vi "Is Calling VI Running.vi"(8 "Error In":errorcluster, 11 "Calling VI Path":path) -> (0 "Error Out":errorcluster, 3 "Running?":bool)   [LabVIEW 2021, in "Notebook.lvlib"]
uses:
  Notebook.lvlib
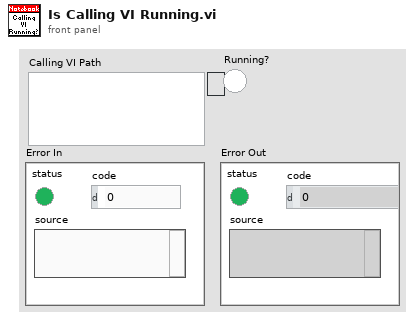
[diagram p1: front panel]
types:
  T1 = enum32{"Bad", "Idle", "Run top level", "Running"}[]
  T2 = enum32{"Invalid", "Standard", "Closed", "Hidden", "Minimized", "Maximized"}[]
  T3 = enum32{"Invalid", "Standard", "Closed", "Hidden", "Minimized", "Maximized"}
  T4 = enum32{"Bad", "Idle", "Run top level", "Running"}
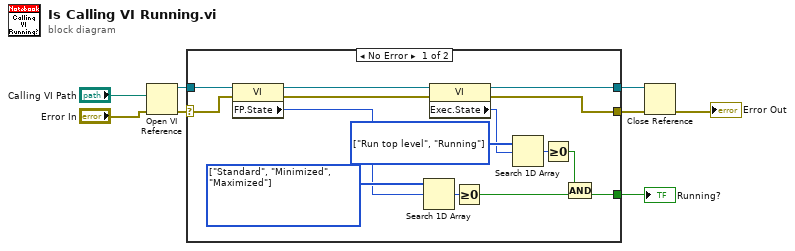
[diagram p0: block diagram]
diagram:
  n1 = Open VI Reference(vi path="Calling VI Path", error in (no error)="Error In") -> (vi reference=w8:refnum<vi>, error out=w6:errorcluster)  [unwired: 4 in]
  n2 = case shown="No Error" w6 {
    selector: w6 -> [w22 w24]
    tunnel: w8 -> [w23 w25]
    tunnel: [w14 w25] -> w7
    tunnel: [w16 w24] -> w5
    tunnel: [w10 _] -> w3
    frame No Error {
      w12 = T1 [enum."Run top level", enum."Running"] items=["Bad", "Idle", "Run top level", "Running"] ("Execution:State")
      w20 = T2 [enum."Standard", enum."Minimized", enum."Maximized"] items=["Invalid", "Standard", "Closed", "Hidden", "Minimized", "Maximized"] ("Front Panel Window:State")
      n3 = property class="VI"(reference=w23, error in=w22) -> (reference out=w15:refnum<vi>, error out=w21:errorcluster, "FP.State"=w19:T3)
      n4 = Search 1D Array(1D array=w20, element=w19) -> (index of element=w18:i32)  [unwired: 1 in]
      n5 = property class="VI"(reference=w15, error in=w21) -> (reference out=w14:refnum<vi>, error out=w16:errorcluster, "Exec.State"=w11:T4)
      n6 = Greater Or Equal To 0?(x=w18) -> (x >= 0?=w17:bool)
      n7 = Search 1D Array(1D array=w12, element=w11) -> (index of element=w13:i32)  [unwired: 1 in]
      n8 = Greater Or Equal To 0?(x=w13) -> (x >= 0?=w9:bool)
      n9 = Compound Arithmetic op=AND(w9, w17) -> (w10:bool)
    }
    frame Error {
    }
  }
  "Running?" <- w3
  n10 = Close Reference(reference=w7, error in (no error)=w5) -> (error out=→"Error Out":errorcluster)
